vi "Create or Open RSA Key.vi"(5 "Key Length (2048)":i32=2048, 6 "Machine Key?":bool, 7 "Crypto Provider":T1, 8 "error in (no error)":errorcluster, 9 "Key Usage (all usages)":i32(ring)=16777215 items=["None"=0, "Decryption"=1, "Signing"=2, "KeyAgreement"=4, "AllUsages"=16777215], 10 "Export Policy (allow export)":i32(ring)=1 items=["None"=0, "AllowExport"=1, "AllowPlaintextExport"=2, "AllowArchiving"=4, "AllowPlaintextArchiving"=8], 11 "Key Name":string) -> (0 "error out":errorcluster, 3 ".NET Refnum out":refnum<k24>)   [LabVIEW 2021, in "dotNET Crypto Key Management.lvlib"]
uses:
  dotNET Crypto Key Management.lvlib
  CNG Provider Type.ctl
  System.Core
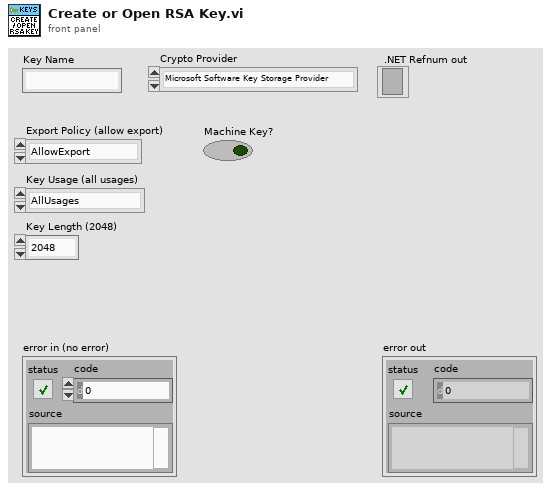
[diagram p1: front panel]
types:
  T1 = typedef "dotNET Crypto Key Management.lvlib/CNG Provider Type.ctl" = enum16{"Microsoft Software Key Storage Provider", "Microsoft Platform Crypto Provider"}
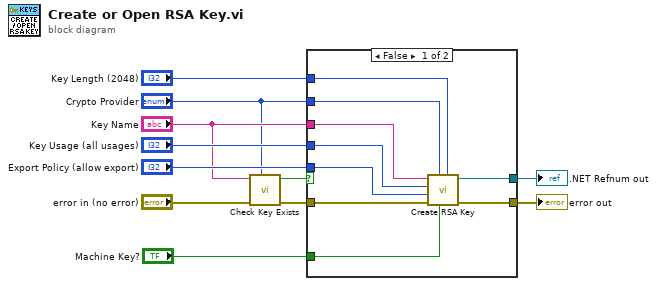
[diagram p0: block diagram]
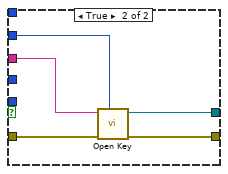
[diagram p2: hidden frame]
diagram:
  n1 = call "Check Key Exists.vi"("Crypto Provider"="Crypto Provider", "error in (no error)"="error in (no error)", "Key Name"="Key Name") -> ("error out"=w4:errorcluster, "Key Exists?"=w1:bool)  [unwired: 7 in]
  n2 = case shown="False" w1 {
    tunnel: [w20 w21] -> w11
    tunnel: [w19 w24] -> w10
    tunnel: "Key Length (2048)" -> [w18 _]
    tunnel: "Machine Key?" -> [w17 _]
    tunnel: "Key Usage (all usages)" -> [w16 _]
    tunnel: "Export Policy (allow export)" -> [w15 _]
    tunnel: w4 -> [w14 w25]
    tunnel: "Key Name" -> [w13 w23]
    tunnel: "Crypto Provider" -> [w12 w22]
    frame False {
      n3 = call "Create RSA Key.vi"("Key Length (2048)"=w18, "Machine Key?"=w17, "Crypto Provider"=w12, "error in (no error)"=w14, "Export Policy (allow export)"=w15, "Key Usage (all usages)"=w16, "Key Name"=w13) -> ("error out"=w19:errorcluster, "CngKey out"=w20:refnum<k24>)  [unwired: 3 in]
    }
    frame True {
      n4 = call "Open Key.vi"("Crypto Provider"=w22, "error in (no error)"=w25, "Key Name"=w23) -> ("error out"=w24:errorcluster, "CngKey out"=w21:refnum<k24>)  [unwired: 7 in]
    }
  }
  ".NET Refnum out" <- w11
  "error out" <- w10
